vi "practica111.vi"() -> ()   [LabVIEW 2013]
uses:
  <vilib>/Native 3D Graph/xcontrol/3DPC_SurfacePlot.xctl
panel:
  out "3D Graph":refnum<class "Base Datatype.lvclass">[](xcontrol)
  out "S2 x":dbl
  out "S2 y":dbl
  out "S1 x":dbl
  out "S1 y":dbl
  in  "S2":i32
  in  "S1":i32
  in  "stop":bool
  in  "S2":dbl(knob) scale=-175.0..175.0
  in  "S1":dbl(knob) scale=0.0..360.0
  out "XY Graph":cluster{"Y":dbl[], "Y":dbl[]}[](graph)
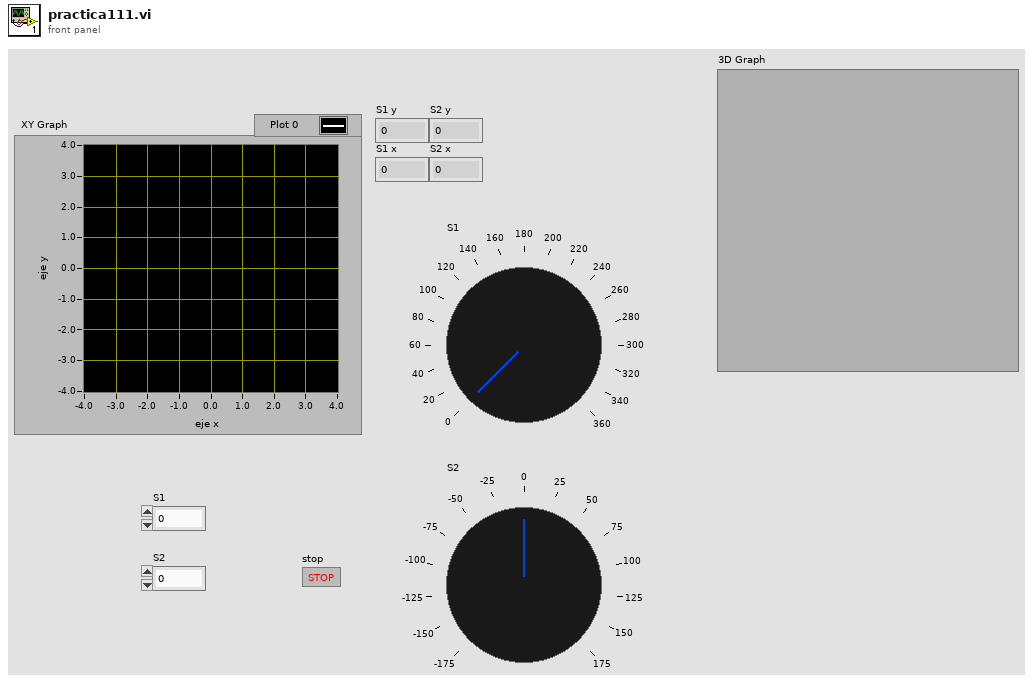
[diagram p1: front panel]
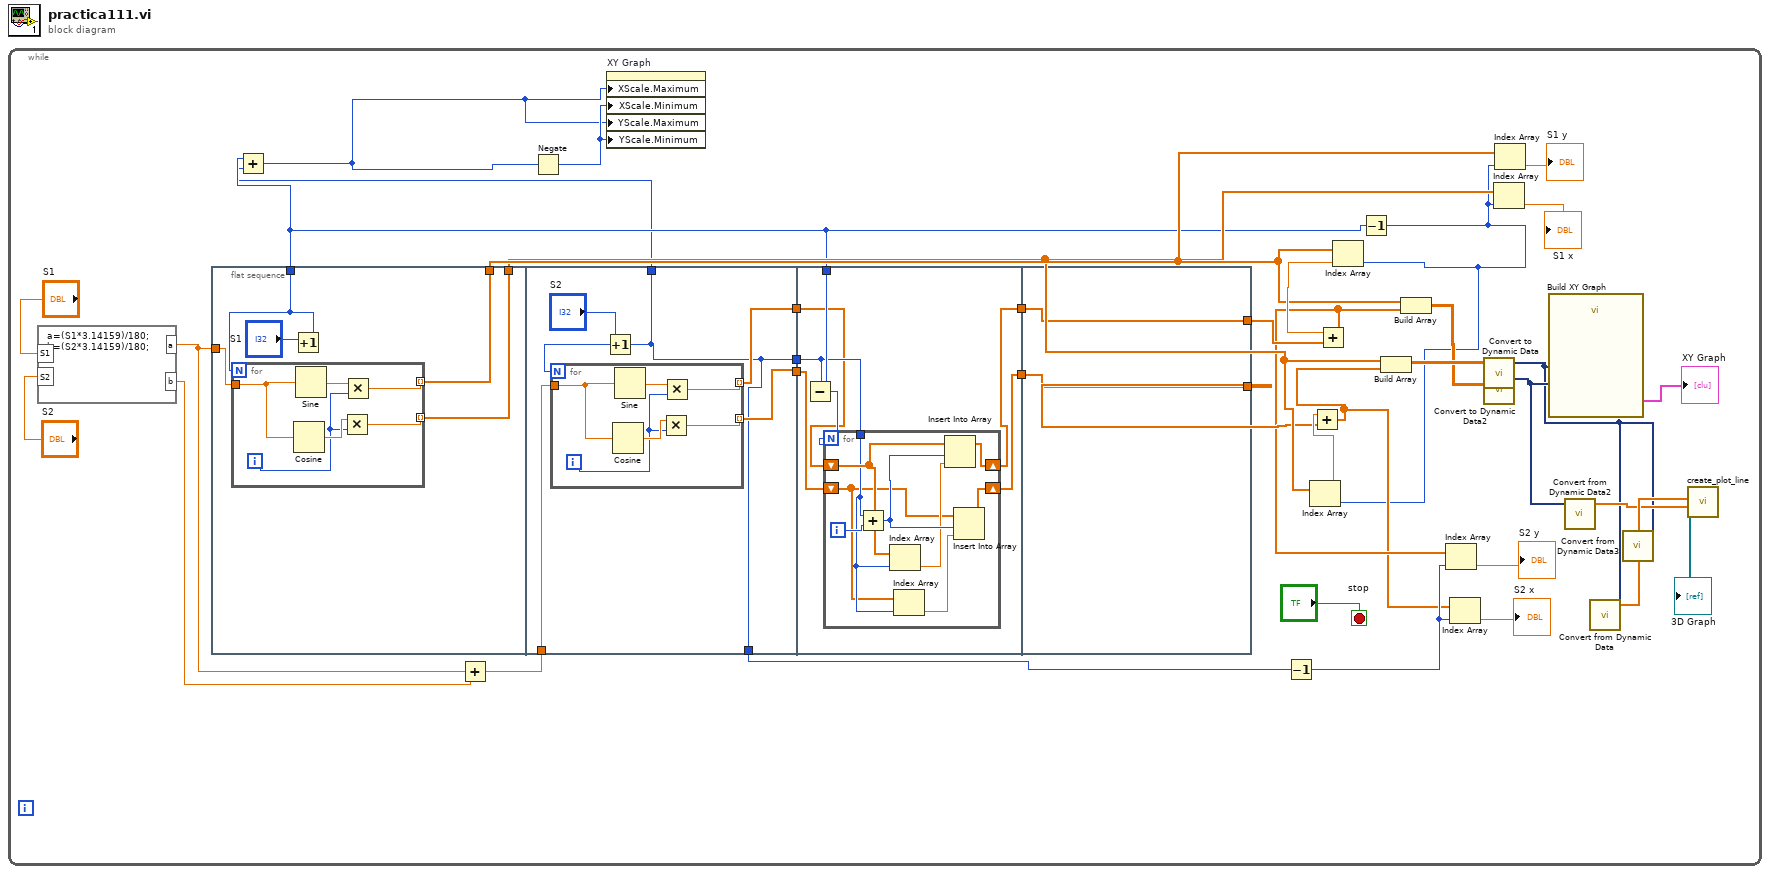
[diagram p0: block diagram]
diagram:
  n1 = while {
    stop <- "stop" stop-if-true
    n2 = formula code="a=(S1*3.14159)/180;\nb=(S2*3.14159)/180;"("S1"="S1", "S2"="S2") -> ("b"=w31:dbl, "a"=w30:dbl)
    n3 = flat-sequence {
      tunnel: w30 -> [w43]
      tunnel: [w39] -> w12
      tunnel: [w41] -> w24
      tunnel: [w40] -> w23
      tunnel: w29 -> [w53]
      tunnel: [w52] -> w27
      tunnel: [w51] -> w26
      tunnel: [w50] -> w25
      tunnel: [w50] -> w15
      tunnel: [w50] -> w11
      tunnel: w27 -> [w61]
      tunnel: w26 -> [w62]
      tunnel: w12 -> [w67]
      tunnel: w25 -> [w65]
      tunnel: [w63] -> w2
      tunnel: [w64] -> w1
      tunnel: [w77] -> w20
      tunnel: [w78] -> w17
      tunnel: w2 -> [w78]
      tunnel: w1 -> [w77]
      frame #0 {
        n4 = Increment(x="S1") -> (x+1=w39:i32)
        n5 = for {
          N: w39 -> [_]
          tunnel: w43 -> [w45]
          tunnel: [w47] -> w41 mode=indexing
          tunnel: [w46] -> w40 mode=indexing
          i -> [w44]
          n6 = Cosine(x=w45) -> (cos(x)=w49:dbl)
          n7 = Sine(x=w45) -> (sin(x)=w48:dbl)
          n8 = Multiply(x=w49, y=w44) -> (x*y=w46:dbl)
          n9 = Multiply(x=w48, y=w44) -> (x*y=w47:dbl)
        }
      }
      frame #1 {
        n10 = Increment(x="S2") -> (x+1=w50:i32)
        n11 = for {
          N: w50 -> [_]
          tunnel: w53 -> [w56]
          tunnel: [w58] -> w51 mode=indexing
          tunnel: [w57] -> w52 mode=indexing
          i -> [w55]
          n12 = Cosine(x=w56) -> (cos(x)=w60:dbl)
          n13 = Sine(x=w56) -> (sin(x)=w59:dbl)
          n14 = Multiply(x=w60, y=w55) -> (x*y=w57:dbl)
          n15 = Multiply(x=w59, y=w55) -> (x*y=w58:dbl)
        }
      }
      frame #2 {
        n16 = Subtract(x=w67, y=w65) -> (x-y=w66:i32)
        n17 = for {
          N: w66 -> [_]
          tunnel: w65 -> [w71]
          shift-right: [w72] -> w64
          shift-left: w62 -> [w74]
          shift-right: [w68] -> w63
          shift-left: w61 -> [w70]
          i -> [w76]
          n18 = Add(x=w71, y=w76) -> (x+y=w75:i32)
          n19 = Index Array(array=w74, index=w71) -> (element=w73:dbl)
          n20 = Index Array(array=w70, index=w71) -> (element=w69:dbl)
          n21 = Insert Into Array(array=w74, index=w75, new element=w73) -> (w72:dbl[])
          n22 = Insert Into Array(array=w70, index=w75, new element=w69) -> (w68:dbl[])
        }
      }
      frame #3 {
      }
    }
    n23 = Add(x=w12, y=w11) -> (x+y=w9:i32)
    n24 = Add(x=w30, y=w31) -> (x+y=w29:dbl)
    n25 = Negate(x=w9) -> (-x=w10:i32)
    n26 = property on="XY Graph" class="XYGraph (strict)"("XScale.Maximum"=w9, "XScale.Minimum"=w10, "YScale.Maximum"=w9, "YScale.Minimum"=w10) -> ()  [unwired: 2 in, 2 out]
    n27 = Decrement(x=w15) -> (x-1=w16:i32)
    n28 = Decrement(x=w12) -> (x-1=w3:i32)
    n29 = Index Array(array=w23, index=w3) -> (element=w32:dbl)
    n30 = Add(x=w32, y=w17) -> (x+y=w13:dbl[])
    n31 = Index Array(array=w24, index=w3) -> (element=w28:dbl)
    n32 = Add(x=w28, y=w20) -> (x+y=w14:dbl[])
    n33 = Build Array(w23, w13) -> (w35:dbl[][])
    n34 = Build Array(w24, w14) -> (w34:dbl[][])
    n35 = Index Array(array=w14, index=w16) -> (element=→"S2 y":dbl)
    n36 = Index Array(array=w13, index=w16) -> (element=→"S2 x":dbl)
    n37 = call "Convert to Dynamic Data"("2D Array"=w35) -> ("Dynamic Data Type"=w4:dynamicdata)  [unwired: 3 in]
    n38 = call "Convert to Dynamic Data2"("2D Array"=w34) -> ("Dynamic Data Type"=w6:dynamicdata)  [unwired: 3 in]
    n39 = Index Array(array=w23, index=w3) -> (element=→"S1 x":dbl)
    n40 = Index Array(array=w24, index=w3) -> (element=→"S1 y":dbl)
    n41 = call "Build XY Graph"("Y Input"=w6, "X Input"=w4) -> ("XY Graph"=→"XY Graph":cluster{"X":dbl[], "Y":dbl[]}[])  [unwired: 8 in, 1 out]
    n42 = call "Convert from Dynamic Data2"("Dynamic Data Type"=w6) -> ("Array"=w5:dbl[])  [unwired: 3 in]
    n43 = call "Convert from Dynamic Data"("Dynamic Data Type"=w4) -> ("Array"=w7:dbl[])  [unwired: 3 in]
    n44 = call "Convert from Dynamic Data3"("Dynamic Data Type"=w4) -> ()  [unwired: 3 in, 1 out]
    n45 = call <vilib>:"create_plot_line.vi"("y vector"=w5, "x vector"=w7) -> ("plots out"=→"3D Graph":refnum<class "Base Datatype.lvclass">[])  [unwired: 3 in, 6 out]
  }
